vi "CreateClass.vi"(8 "error in (no error)":errorcluster, 11 "GenLVOOP in":refnum<class "GenLVOOP.lvclass">) -> (0 "error out":errorcluster, 3 "GenLVOOP out":refnum<class "GenLVOOP.lvclass">)   [LabVIEW 2013, in "GenLVOOP.lvclass"]
uses:
  GenLVOOP.lvclass
  ProjectHandler/RefNums.vi
  ProjectHandler.lvlib
  baseClass/baseClass.lvclass
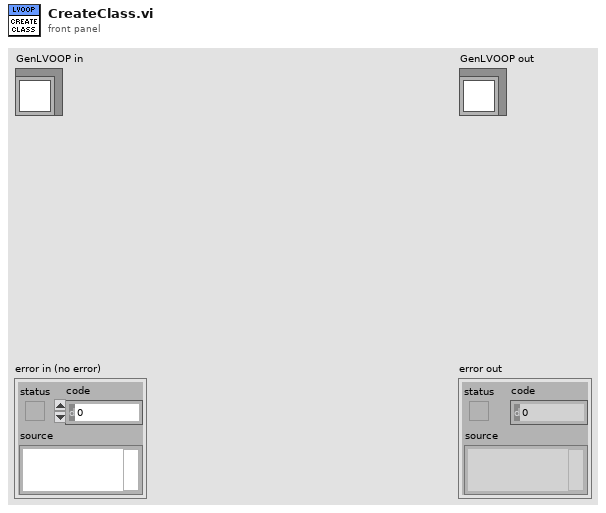
[diagram p1: front panel]
types:
  T1 = cluster{"App":refnum<vi>, "Project":refnum<vi>, "My Computer":refnum<vi>}
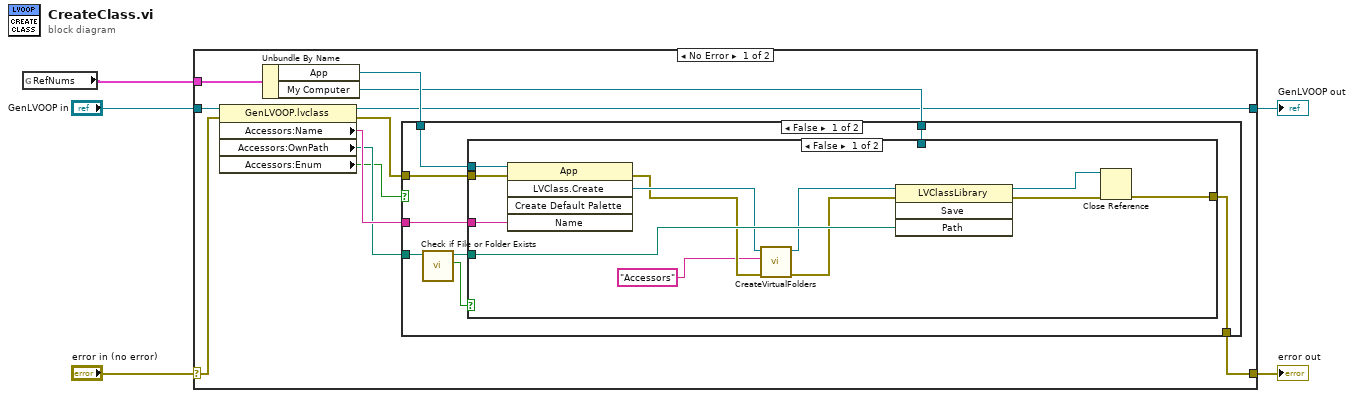
[diagram p0: block diagram]
diagram:
  n1 = global read "RefNums.vi" "RefNums"() -> (w1:T1)
  n2 = case shown="No Error" "error in (no error)" {
    selector: "error in (no error)" -> [w9 w39]
    tunnel: [w10 w39] -> w4
    tunnel: [w6 w38] -> w2
    tunnel: "GenLVOOP in" -> [w16 w38]
    tunnel: w1 -> [w8 _]
    frame No Error {
      n3 = property class="GenLVOOP.lvclass"(reference=w16, error in=w9) -> (reference out=w6:refnum<class "GenLVOOP.lvclass">, error out=w14:errorcluster, "Accessors:Name"=w13:string, "Accessors:OwnPath"=w12:path, "Accessors:Enum"=w7:bool)
      n4 = Unbundle By Name(w8) -> ("App"=w15:refnum<vi>, "My Computer"=w11:refnum<vi>)
      n5 = case shown="False" w7 {
        tunnel: w15 -> [w23 _]
        tunnel: w14 -> [w22 w37]
        tunnel: w13 -> [w21 _]
        tunnel: w12 -> [w20 _]
        tunnel: w11 -> [w19 _]
        tunnel: [w18 w37] -> w10
        frame False {
          n6 = call <vilib>:"Check if File or Folder Exists.vi"("path"=w20) -> ("file or folder exists?"=w17:bool)  [unwired: 8 in, 2 out]
          n7 = case shown="False" w17 {
            tunnel: w23 -> [w35 _]
            tunnel: w22 -> [w34 w36]
            tunnel: w21 -> [w33 _]
            tunnel: w20 -> [w32 _]
            tunnel: w19 -> [_ _]
            tunnel: [w30 w36] -> w18
            frame False {
              n8 = invoke class="App" method="LVClass.Create"(reference=w35, error in=w34, "Name"=w33) -> (error out=w26:errorcluster, "LVClass.Create"=w28:refnum<vi>)  [unwired: 2 in, 3 out]
              n9 = call "CreateVirtualFolders.vi"("error in (no error)"=w26, "Name"="Accessors", "LabVIEW Class In"=w28) -> ("error out"=w25:errorcluster, "LabVIEW Class Out"=w27:refnum<vi>)  [unwired: 7 in]
              n10 = invoke class="LVClassLibrary" method="Save"(reference=w27, error in=w25, "Path"=w32) -> (reference out=w31:refnum<vi>, error out=w29:errorcluster)  [unwired: 1 in, 2 out]
              n11 = Close Reference(reference=w31, error in (no error)=w29) -> (error out=w30:errorcluster)
            }
            frame True {
            }
          }
        }
        frame True {
        }
      }
    }
    frame Error {
    }
  }
  "error out" <- w4
  "GenLVOOP out" <- w2
